vi "Configure GB Test Time.vi"(8 "error in (no error)":errorcluster, 9 "Test Time [s]":dbl=3.0 min=0.0 max=999.0 step=0.1 format="%.1f", 10 "Step":T1=1 min=1 max=99 step=1, 11 "VISA resource name":refnum<visa-resource-name>) -> (0 "error out":errorcluster, 3 "VISA resource name out":refnum<visa-resource-name>)   [LabVIEW 2025, in "Chroma 19572.lvlib"]
uses:
  <instrlib>/Chroma 19572/Chroma 19572.lvlib
  <instrlib>/Chroma 19572/Public/Utility/Type Def/steps--numeric.ctl
panel:
  # "Configure GB Test Time"
  # "0=CONT.\n0,5 to 999 sec"
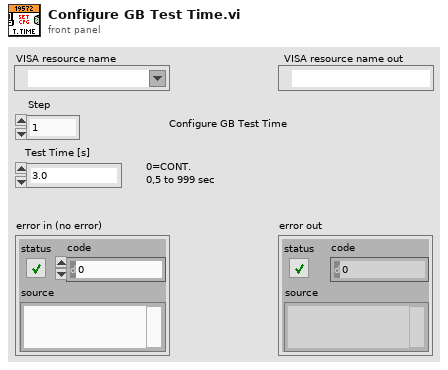
[diagram p1: front panel]
types:
  T1 = typedef "Chroma 19572.lvlib/steps--numeric.ctl" = u8
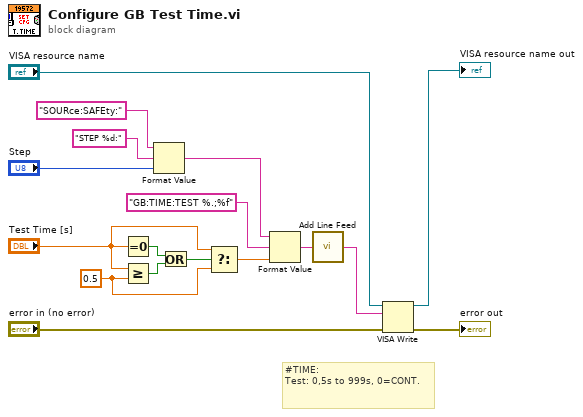
[diagram p0: block diagram]
diagram:
  w4 = 0.5 ("y")
  # "#TIME: \nTest: 0,5s to 999s, 0=CONT."
  n1 = Equal To 0?(x="Test Time [s]") -> (x = 0?=w7:bool)
  n2 = Greater Or Equal?(x="Test Time [s]", y=w4) -> (x >= y?=w6:bool)
  n3 = Format Value(string ("")="SOURce:SAFEty:", format string="STEP %d:", value (0)="Step") -> (output string=w1:string)
  n4 = Or(x=w7, y=w6) -> (x .or. y?=w5:bool)
  n5 = Select(t="Test Time [s]", s=w5, f=w4) -> (s? t:f=w2:dbl)
  n6 = Format Value(string ("")=w1, format string="GB:TIME:TEST %.;%f", value (0)=w2) -> (output string=w13:string)
  n7 = call <instrlib>:"Add Line Feed.vi"("Command string"=w13) -> ("Concatenated string"=w12:string)  [unwired: 4 in]
  n8 = VISA Write(VISA resource name="VISA resource name", write buffer=w12, error in (no error)="error in (no error)") -> (VISA resource name out=→"VISA resource name out":refnum<visa-resource-name>, error out=→"error out":errorcluster)  [unwired: 1 out]
